vi "Write SampleDataArray.vi"(8 "error in (no error)":errorcluster, 10 "SampleDataArray":T1 {"Timestamp" format="%.6f"}, 11 "AnalysisPluginsBase in":refnum<class "AnalysisPluginsBase.lvclass">) -> (0 "error out":errorcluster, 3 "AnalysisPluginsBase out":refnum<class "AnalysisPluginsBase.lvclass">)   [LabVIEW 2014]
uses:
  AnalysisPluginsBase.lvclass
  Typedefs/clSampleData.ctl
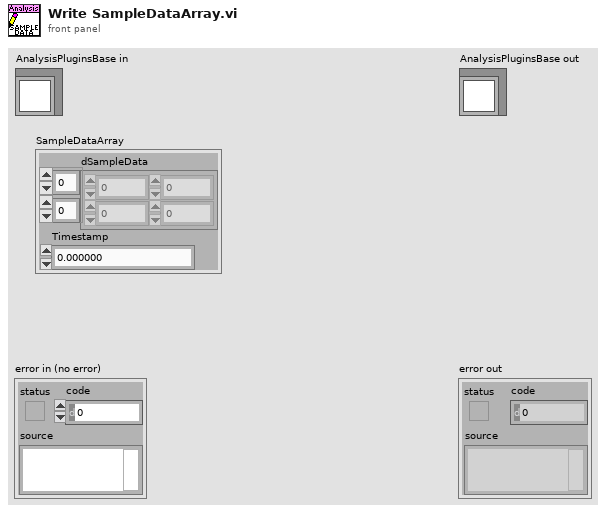
[diagram p1: front panel]
types:
  T1 = typedef "AnalysisPlugins.lvlib/AnalysisPluginsBase.lvclass/clSampleData.ctl" = cluster{"dSampleData":dbl[][], "Timestamp":ext}
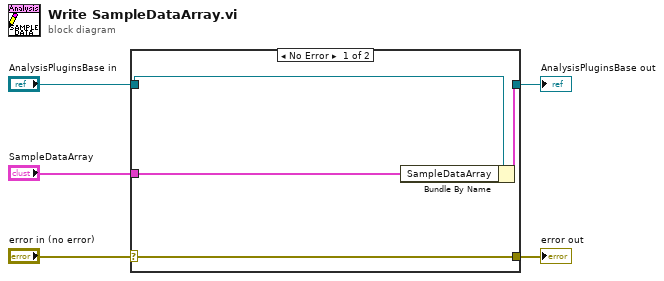
[diagram p0: block diagram]
diagram:
  n1 = case shown="No Error" "error in (no error)" {
    selector: "error in (no error)" -> [w9 w10]
    tunnel: [w9 w10] -> w4
    tunnel: [w7 w11] -> w2
    tunnel: "AnalysisPluginsBase in" -> [w8 w11]
    tunnel: "SampleDataArray" -> [w6 _]
    frame No Error {
      n2 = Bundle By Name(cluster=w8, "SampleDataArray"=w6) -> (w7:cluster{})
    }
    frame Error {
    }
  }
  "error out" <- w4
  "AnalysisPluginsBase out" <- w2
